vi "Main.vi"() -> ()   [LabVIEW 2019, in "TestDataMarshal.lvlib" / "TestDataMarshal.lvclass"]
uses:
  TestDataMarshal.lvclass
  typeDefs/Server State Data.ctl
  TestDataMarshal.lvclass/TestDataMarshal.ctl
panel:
  out "Listening Port":i32
  in  "Stop":bool
  in  "Enable Async Mode":bool
  in  "Server Address":string="0.0.0.0:50051"
  in  "Server Certificate File (.crt)":path
  in  "Server Key File (.key)":path
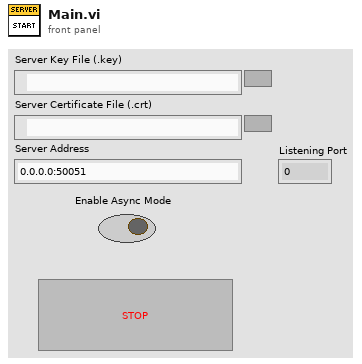
[diagram p1: front panel]
types:
  T1 = typedef "TestDataMarshal.lvlib/TestDataMarshal.lvclass/Server State Data.ctl" = cluster{"Data":string}
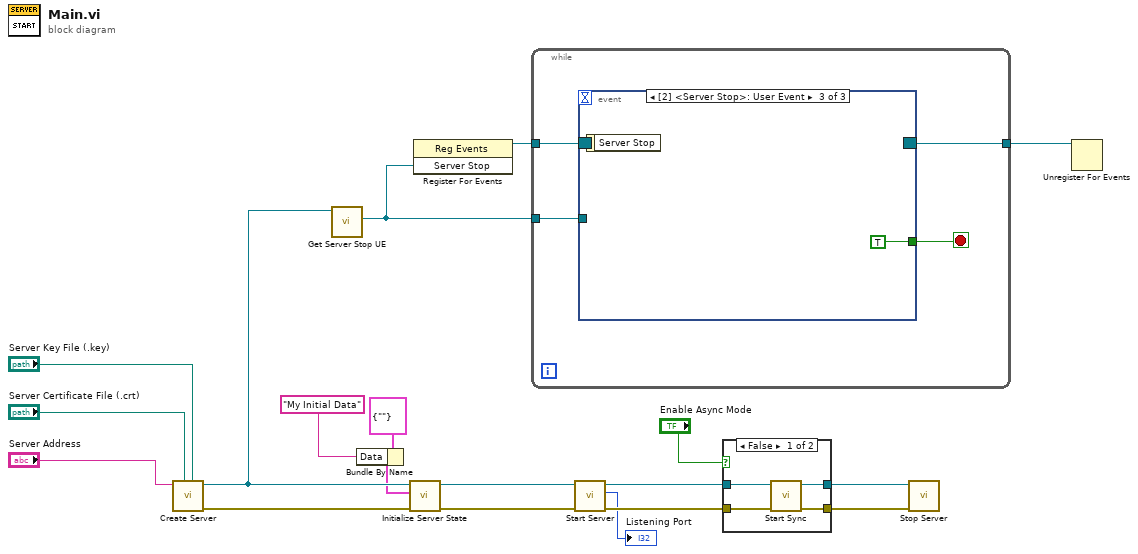
[diagram p0: block diagram]
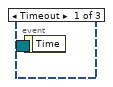
[diagram p2: hidden frame]
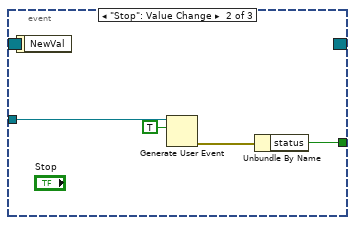
[diagram p3: hidden frame]
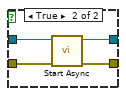
[diagram p4: hidden frame]
diagram:
  n1 = call "Create Server.vi"("Server Key File (.key)"="Server Key File (.key)", "Server Certificate File (.crt)"="Server Certificate File (.crt)", "Server Address"="Server Address") -> ("error out"=w8:errorcluster, "gRPC Server out"=w5:refnum<class "TestDataMarshal.lvclass">)  [unwired: 7 in]
  n2 = call "Get Server Stop UE.vi"("OOP Server in"=w5) -> ("Server Stop"=w9:refnum<user-event>)  [unwired: 9 in, 1 out]
  n3 = Bundle By Name(cluster=T1 {"Data"=""} ("Initial State"), "Data"="My Initial Data") -> (w3:T1)
  n4 = call "Initialize Server State.vi"("error in (no error)"=w8, "Initial State"=w3, "gRPC Server in"=w5) -> ("error out"=w7:errorcluster, "gRPC Server out"=w6:refnum<class "TestDataMarshal.lvclass">)  [unwired: 7 in]
  n5 = register-events(w9) -> (reference out=w11:refnum<event-registration>)  [unwired: 2 in, 1 out]
  n6 = while {
    tunnel: w9 -> [w23]
    tunnel: w11 -> [w22]
    tunnel: [w20] -> w10
    stop <- w21 stop-if-true
    n7 = event shown="[2] <Server Stop>: User Event" {
      selector: w22 -> [_ _ _]
      dyn-events: [_ _ _] -> w20
      timeout: _ -> [_ _ _]
      tunnel: w23 -> [_ w27 _]
      tunnel: [_ w24 TRUE] -> w21
      event Timeout {
        n8 = event-data() -> ()  [unwired: 1 in, 1 out]
      }
      event "Stop": Value Change {
        n9 = event-data() -> ()  [unwired: 1 in, 1 out]
        n10 = Generate User Event(user event=w27, event data cluster=TRUE ("event data")) -> (error out=w25:errorcluster)  [unwired: 2 in, 1 out]
        n11 = Unbundle By Name(w25) -> ("status"=w24:bool)
      }
      event User Event {
        n12 = event-data() -> ()  [unwired: 1 in, 1 out]
      }
    }
  }
  n13 = call "Start Server.vi"("error in (no error)"=w7, "gRPC Server in"=w6) -> ("error out"=w19:errorcluster, "Listening Port"=→"Listening Port":i32, "gRPC Server out"=w18:refnum<class "TestDataMarshal.lvclass">)  [unwired: 7 in]
  n14 = case shown="False" "Enable Async Mode" {
    tunnel: w19 -> [w32 w36]
    tunnel: w18 -> [w31 w35]
    tunnel: [w30 w33] -> w17
    tunnel: [w29 w34] -> w16
    frame False {
      n15 = call "Start Sync.vi"("error in (no error)"=w32, "gRPC Server in"=w31) -> ("error out"=w30:errorcluster, "gRPC Server out"=w29:refnum<class "TestDataMarshal.lvclass">)  [unwired: 8 in]
    }
    frame True {
      n16 = call "Start Async.vi"("error in (no error)"=w36, "gRPC Server in"=w35) -> ("error out"=w33:errorcluster, "gRPC Server out"=w34:refnum<class "TestDataMarshal.lvclass">)  [unwired: 8 in]
    }
  }
  n17 = call "Stop Server.vi"("error in (no error)"=w17, "gRPC Server in"=w16) -> ()  [unwired: 9 in, 1 out]
  n18 = Unregister For Events(event registration refnum=w10) -> ()  [unwired: 1 in, 1 out]
